vi "Read Plugin Group IDs.vi"(8 "error in (no error)":errorcluster, 10 "plugin ID":string, 11 "Configuration Session":refnum<class "Configuration Session.lvclass">) -> (0 "error out":errorcluster, 1 "group IDs":string[](array[string]), 3 "Configuration Session out":refnum<class "Configuration Session.lvclass">, 4 "found?":bool)   [LabVIEW 2017, in "DSF Core.lvlib" / "Configuration Session.lvclass"]
uses:
  Configuration Session.lvclass
  Configuration Session.lvclass/Configuration Session.ctl
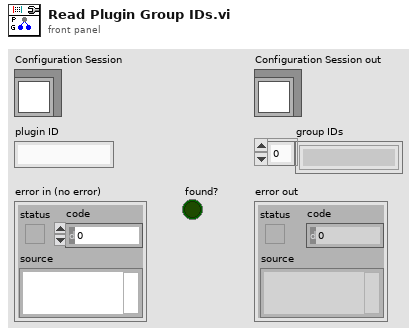
[diagram p1: front panel]
types:
  T1 = typedef "DSF Core.lvlib/Configuration Session.lvclass/DSF Config Data Ref.ctl" = refnum<data-value>
  T2 = typedef "DSF Core.lvlib/Configuration Session.lvclass/DSF Config Data.ctl" = cluster{"dsf configuration":T3, "path":path, "dirty":bool}
  T3 = typedef "DSF Core.lvlib/Configuration Session.lvclass/Internal DSF Configuration.ctl" = cluster{"dsfversion":T4, "version":T4, "plugins":T5[], "groups":T8[], "transfers":T10[], "channels":T12[], "settings":T14[]}
  T4 = typedef "DSF Core.lvlib/DSF Version Info.ctl" = cluster{"major":u32, "minor":u32, "fix":u32, "build":string}
  T5 = typedef "DSF Core.lvlib/Configuration Session.lvclass/Internal DSF Plugin with ID.ctl" = cluster{"id":string, "values":T6}
  T6 = typedef "DSF Core.lvlib/Configuration Session.lvclass/Internal DSF Plugin Info.ctl" = cluster{"type":string, "timing":T7, "group ids":string[], "settings id":string, "thread count":i32}
  T7 = typedef "DSF Core.lvlib/DSF Timing Info.ctl" = cluster{"priority":u64, "decimation":u64, "offset":u64}
  T8 = typedef "DSF Core.lvlib/Configuration Session.lvclass/Internal DSF Group with ID.ctl" = cluster{"id":string, "values":T9}
  T9 = typedef "DSF Core.lvlib/Configuration Session.lvclass/Internal DSF Group Info.ctl" = cluster{"direction":i32, "timing":T7, "transfer ids":string[], "settings id":string}
  T10 = typedef "DSF Core.lvlib/Configuration Session.lvclass/Internal DSF Transfer with ID.ctl" = cluster{"id":string, "values":T11}
  T11 = typedef "DSF Core.lvlib/Configuration Session.lvclass/Internal DSF Transfer Info.ctl" = cluster{"byte order":i32, "channel ids":string[], "settings id":string}
  T12 = typedef "DSF Core.lvlib/Configuration Session.lvclass/Internal DSF Channel with ID.ctl" = cluster{"id":string, "values":T13}
  T13 = typedef "DSF Core.lvlib/Configuration Session.lvclass/Internal DSF Channel Info.ctl" = cluster{"count":u64, "buffer offset":u64, "data type":i32, "settings id":string}
  T14 = typedef "DSF Core.lvlib/Configuration Session.lvclass/Internal DSF Settings with ID.ctl" = cluster{"id":string, "values":T15}
  T15 = typedef "DSF Core.lvlib/Configuration Session.lvclass/Internal DSF Settings Info.ctl" = cluster{"key":string, "value":string}[]
  T16 = typedef "DSF Core.lvlib/DSF Plugin Info.ctl" = cluster{"type":string, "timing":T7, "group ids":string[], "settings id":string, "thread count":i32}
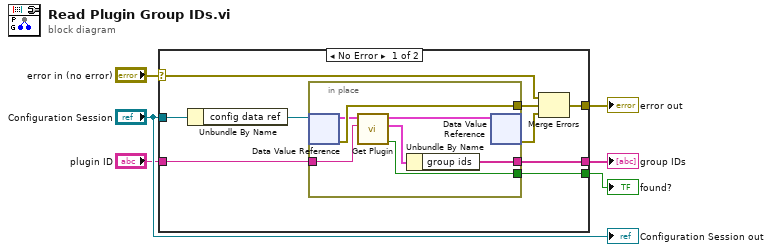
[diagram p0: block diagram]
diagram:
  n1 = case shown="No Error" "error in (no error)" {
    selector: "error in (no error)" -> [w15 w23]
    tunnel: "Configuration Session" -> [w8 _]
    tunnel: [w13 w23] -> w4
    tunnel: "plugin ID" -> [w14 _]
    tunnel: [w11 _] -> w2
    tunnel: [w10 _] -> w1
    frame No Error {
      n2 = Unbundle By Name(w8) -> ("config data ref"=w7:T1)
      n3 = in-place {
        in-place-border: w14 -> [w22]
        in-place-border: [w21] -> w11
        in-place-border: [w19] -> w10
        in-place-border: [w18] -> w9
        n4 = in-place-dvr #1(w7) -> (w16:T2, w18:errorcluster)
        n5 = call "Get Plugin.vi"("id"=w22, "DSF Configuration in"=w16) -> ("exists?"=w21:bool, "info"=w20:T16, "DSF Configuration out"=w17:T2)  [unwired: 6 in, 1 out]
        n6 = Unbundle By Name(w20) -> ("group ids"=w19:string[])
        n7 = in-place-dvr #1(w17) -> (w12:errorcluster)  [unwired: 1 out]
      }
      n8 = Merge Errors(w15, w9, w12) -> (w13:errorcluster)
    }
    frame Error {
    }
  }
  "error out" <- w4
  "found?" <- w2
  "group IDs" <- w1
  "Configuration Session out" <- "Configuration Session"
